vi "Set Columns.vi"(3 "error in (no error)":errorcluster, 4 "Columns in":refnum<class "Column.lvclass">[](array[class]), 5 "Pulseblaster in":refnum<class "Pulseblaster.lvclass">) -> (0 "error out":errorcluster, 1 "Pulseblaster out":refnum<class "Pulseblaster.lvclass">)   [LabVIEW 2013, in "Pulseblaster.lvclass"]
uses:
  Pulseblaster.lvclass
  ColumnVIs/Column/Column.lvclass
  <vilib>/Utility/error.llb/DialogType.ctl
  Master Device/Master Device.lvclass
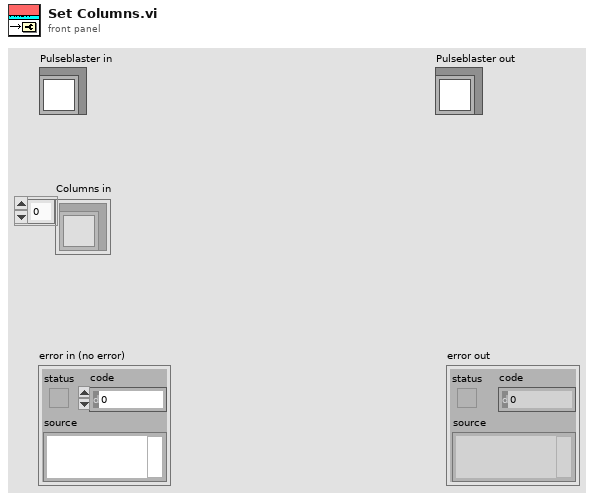
[diagram p1: front panel]
types:
  T1 = typedef "DialogType.ctl" = u16
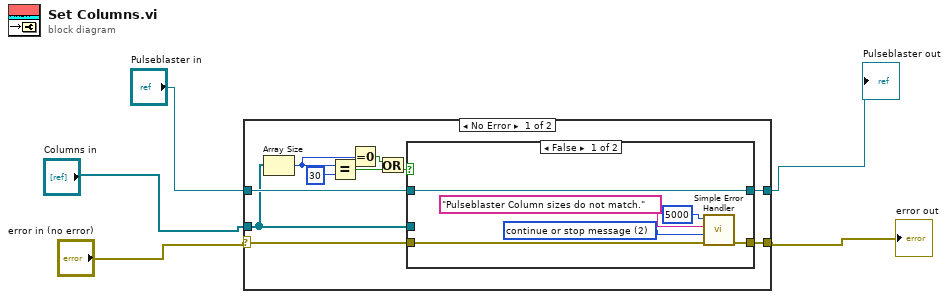
[diagram p0: block diagram]
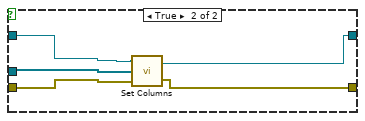
[diagram p2: hidden frame]
diagram:
  n1 = case shown="No Error" "error in (no error)" {
    selector: "error in (no error)" -> [w12 w27]
    tunnel: [w15 w27] -> w2
    tunnel: [w14 w28] -> w1
    tunnel: "Columns in" -> [w11 _]
    tunnel: "Pulseblaster in" -> [w13 w28]
    frame No Error {
      n2 = Array Size(array=w11) -> (size(s)=w6:i32)
      n3 = Equal?(x=w6, y=30) -> (x = y?=w9:bool)
      n4 = Equal To 0?(x=w6) -> (x = 0?=w7:bool)
      n5 = Or(x=w7, y=w9) -> (x .or. y?=w8:bool)
      n6 = case shown="False" w8 {
        tunnel: [w17 w22] -> w15
        tunnel: [w19 w23] -> w14
        tunnel: w11 -> [_ w25]
        tunnel: w13 -> [w19 w26]
        tunnel: w12 -> [w18 w24]
        frame False {
          w20 = T1 2 items=["no dialog", "OK message", "continue or stop message", "OK message + warnings", "continue/stop + warnings"] ("type of dialog (OK msg:1)")
          n7 = call <vilib>:"Simple Error Handler.vi"("error code (no error:0)"=5000, "error source (\" \")"="Pulseblaster Column sizes do not match." ("message"), "type of dialog (OK msg:1)"=w20, "error in (no error)"=w18) -> ("error out"=w17:errorcluster)  [unwired: 1 in, 4 out]
        }
        frame True {
          n8 = call-parent "Set Columns.vi"("error in (no error)"=w24, "Columns"=w25, "Device in"=w26) -> ("error out"=w22:errorcluster, "Device out"=w23:refnum<class "Pulseblaster.lvclass">)  [unwired: 1 in]
        }
      }
    }
    frame Error {
    }
  }
  "error out" <- w2
  "Pulseblaster out" <- w1
